vi "getPath.vi"(0 "reference":refnum<class "GeneralPathEdge.lvclass">, 5 "error in (no error)":errorcluster) -> (14 "reference out":refnum<class "GeneralPathEdge.lvclass">, 15 "points":T1[](array[typedef]) {"y" format="%.2f"; "x" format="%.2f"}, 19 "error out":errorcluster)   [LabVIEW 2012, in "GeneralPathEdge.lvclass"]
doc: "Abstract getPath function"
uses:
  <resource>/Framework/Providers/Open_GDS/UML/GeneralPathEdge_class/GeneralPathEdge.lvclass
  <resource>/Framework/Providers/Open_GDS/UML/General/Point/Point Point2D.ctl
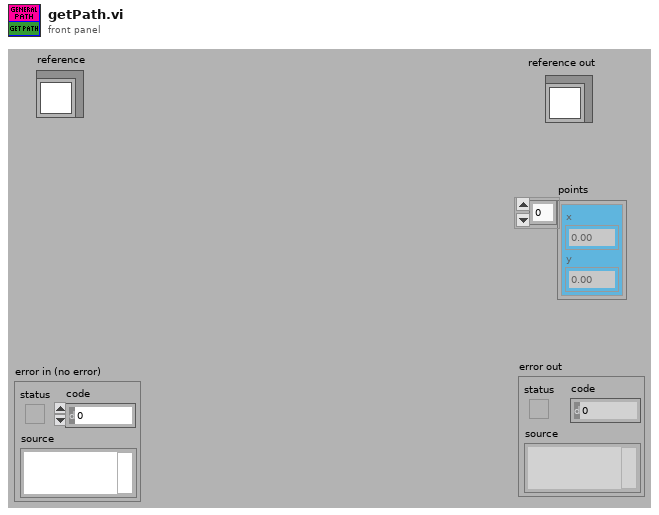
[diagram p1: front panel]
types:
  T1 = typedef "Point Point2D.ctl" = cluster{"x":dbl, "y":dbl}
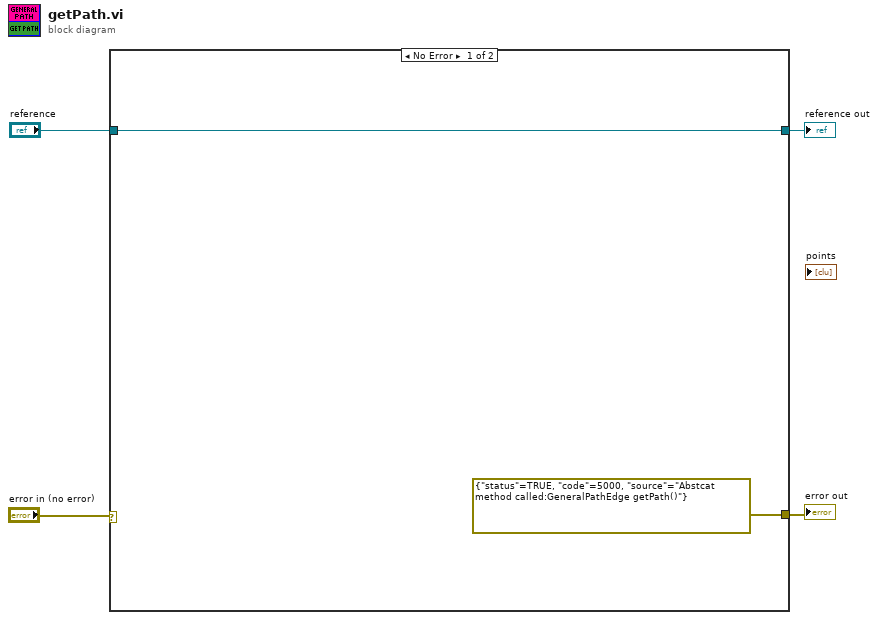
[diagram p0: block diagram]
diagram:
  n1 = case shown="No Error" "error in (no error)" {
    selector: "error in (no error)" -> [_ w7]
    tunnel: "reference" -> [w6 w8]
    tunnel: [errorcluster {"status"=TRUE, "code"=5000, "source"="Abstcat method called:GeneralPathEdge getPath()"} ("error out") w7] -> w3
    tunnel: [w6 w8] -> w2
    frame No Error {
    }
    frame Error {
    }
  }
  "reference out" <- w2
  "error out" <- w3
